vi "MFCStart.vi"(8 "Error In":errorcluster, 11 "VISA Resource List":string[](array[string])) -> (0 "Error Out":errorcluster, 3 "Sierra M100 Out":refnum<visa-resource-name>)   [LabVIEW 2012]
uses:
  MFCConfigurationGlobalAction.ctl
  libs/LV-Utilities/LV-Utilities.lvlib
  libs/Sierra-M100/Sierra-M100.lvlib
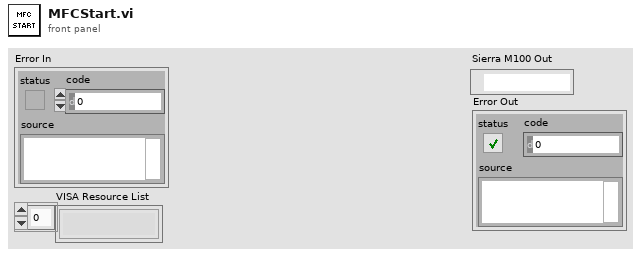
[diagram p1: front panel]
types:
  T1 = typedef "MFCConfigurationGlobalAction.ctl" = enum16{"Init", "Get", "Set", "Add", "Remove", "Reset"}
  T2 = typedef "MFCConfiguration.ctl" = cluster{"COM Port":u32, "Timeout (msec)":u32, "Setpoint":dbl, "Valve State":T3, "Gas":T4, "Units":T5, "Serial Number":string, "Firmware Version":string}
  T3 = typedef "Sierra-M100.lvlib/ValveState.ctl" = enum16{"Automatic", "Closed", "Purge"}
  T4 = typedef "Sierra-M100.lvlib/Gas.ctl" = enum16{"Air", "Argon", "CO2", "CO", "Helium", "Hydrogen", "Methane", "Nitrogen", "Nitrous Oxide", "Oxygen"}
  T5 = typedef "Sierra-M100.lvlib/Units.ctl" = enum16{"scc/s", "scc/m", "scc/H", "Ncc/s", "Ncc/m", "Ncc/H", "SCF/s", "SCF/m", "SCF/H", "NM3/s", "NM3/m", "NM3/H", "SM3/s", "SM3/m", "SM3/H", "sl/s", "sl/m", "sl/H", "NL/s", "NL/m", "Nl/H", "g/s", "g/m", "g/H", "kg/s", "kg/m", "kg/H", "lb/s", "lb/m", "lb/H"}
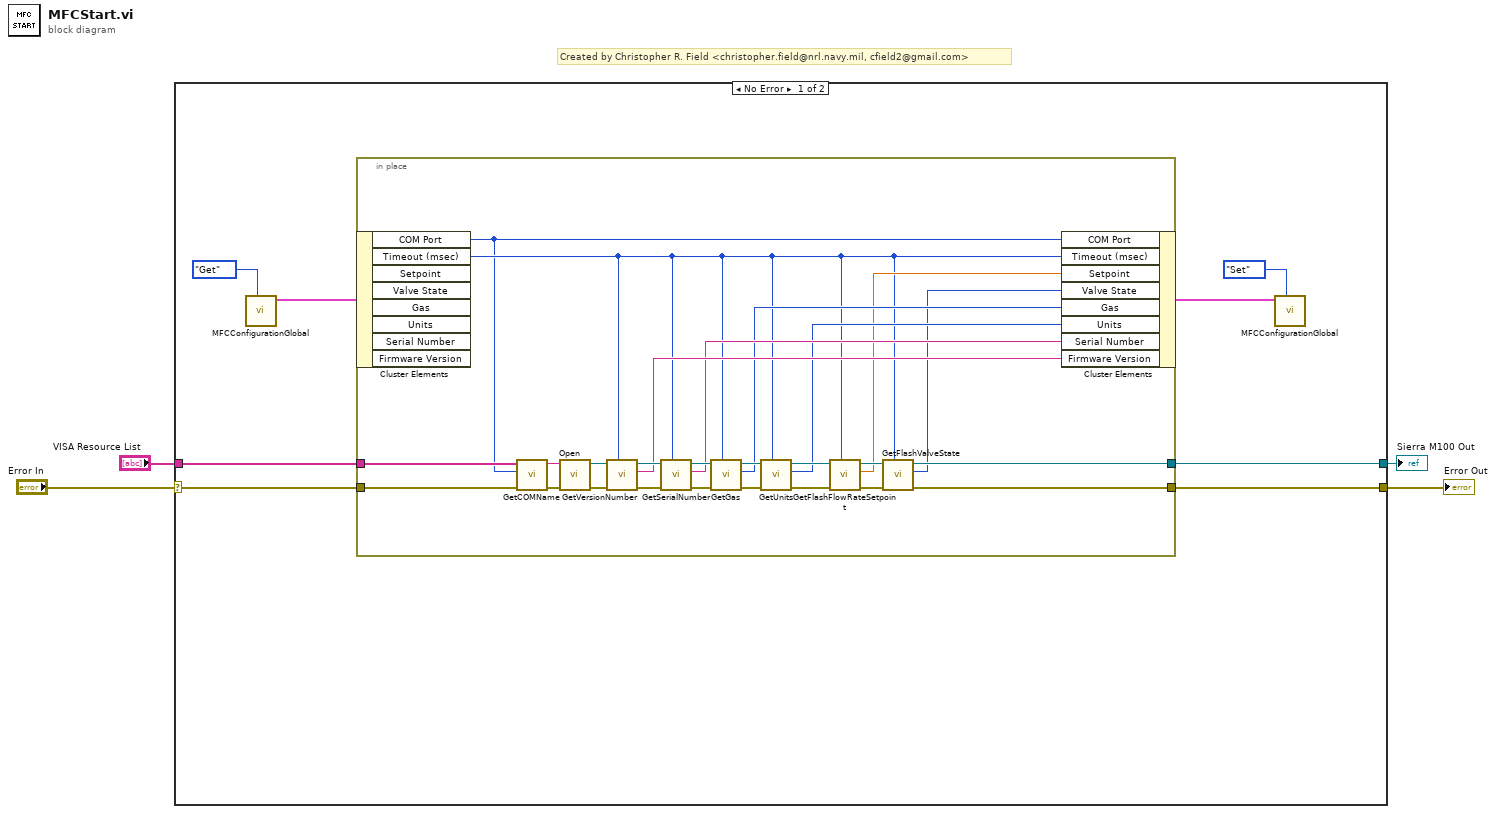
[diagram p0: block diagram]
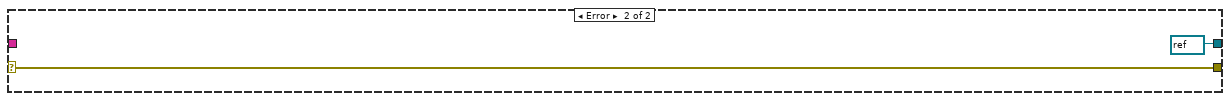
[diagram p2: hidden frame]
diagram:
  # "Created by Christopher R. Field <christopher.field@nrl.navy.mil, cfield2@gmail.com>"
  n1 = case shown="No Error" "Error In" {
    selector: "Error In" -> [w11 w40]
    tunnel: "VISA Resource List" -> [w10 _]
    tunnel: [w8 refnum<visa-resource-name> refnum ("Sierra M100 Out")] -> w2
    tunnel: [w7 w40] -> w1
    frame No Error {
      n2 = call "MFCConfigurationGlobal.vi"("Action"=MFCConfigurationGlobalAction."Get") -> ("Value Out"=w6:T2)  [unwired: 10 in]
      n3 = in-place {
        in-place-border: w11 -> [w28]
        in-place-border: w10 -> [w27]
        in-place-border: [w26] -> w8
        in-place-border: [w25] -> w7
        n4 = in-place-cluster #1(w6) -> ("COM Port"=w13:u32, "Timeout (msec)"=w14:u32)  [unwired: 6 out]
        n5 = call "GetCOMName.vi"("Error In"=w28, "COM Port"=w13, "VISA Resource List"=w27) -> ("Error Out"=w37:errorcluster, "VISA COM Resource Name"=w38:string)  [unwired: 6 in, 1 out]
        n6 = call "Open.vi"("Error In"=w37, "Sierra M100 In"=w38) -> ("Error Out"=w35:errorcluster, "Sierra M100 Out"=w36:refnum<visa-resource-name>)  [unwired: 8 in]
        n7 = call "GetVersionNumber.vi"("Timeout (ms)"=w14, "Error In"=w35, "Sierra M100 In"=w36) -> ("Error Out"=w33:errorcluster, "Version Number"=w20:string, "Sierra M100 Out"=w34:refnum<visa-resource-name>)  [unwired: 6 in]
        n8 = call "GetSerialNumber.vi"("Timeout (ms)"=w14, "Error In"=w33, "Sierra M100 In"=w34) -> ("Error Out"=w31:errorcluster, "Serial Number"=w19:string, "Sierra M100 Out"=w32:refnum<visa-resource-name>)  [unwired: 6 in]
        n9 = call "GetGas.vi"("Timeout (ms)"=w14, "Error In"=w31, "Sierra M100 In"=w32) -> ("Error Out"=w29:errorcluster, "Gas"=w18:T4, "Sierra M100 Out"=w30:refnum<visa-resource-name>)  [unwired: 6 in]
        n10 = call "GetUnits.vi"("Timeout (ms)"=w14, "Error In"=w29, "Sierra M100 In"=w30) -> ("Error Out"=w23:errorcluster, "Units"=w17:T5, "Sierra M100 Out"=w24:refnum<visa-resource-name>)  [unwired: 6 in]
        n11 = call "GetFlashFlowRateSetpoint.vi"("Timeout (ms)"=w14, "Error In"=w23, "Sierra M100 In"=w24) -> ("Error Out"=w22:errorcluster, "Setpoint (mL/min)"=w16:dbl, "Sierra M100 Out"=w21:refnum<visa-resource-name>)  [unwired: 6 in]
        n12 = call "GetFlashValveState.vi"("Timeout (ms)"=w14, "Error In"=w22, "Sierra M100 In"=w21) -> ("Error Out"=w25:errorcluster, "Valve State"=w15:T3, "Sierra M100 Out"=w26:refnum<visa-resource-name>)  [unwired: 6 in]
        n13 = in-place-cluster #1("COM Port"=w13, "Timeout (msec)"=w14, "Setpoint"=w16, "Valve State"=w15, "Gas"=w18, "Units"=w17, "Serial Number"=w19, "Firmware Version"=w20) -> (w5:T2)
      }
      n14 = call "MFCConfigurationGlobal.vi"("Action"=MFCConfigurationGlobalAction."Set", "Set Value"=w5) -> ()  [unwired: 9 in, 1 out]
    }
    frame Error {
    }
  }
  "Sierra M100 Out" <- w2
  "Error Out" <- w1
